vi "Custom - TDD Input Read.vi"(5 "Trigger Offset (dBm)":dbl, 6 "Path Loss (dBm)":dbl, 7 "Sample Count":dbl=16.0, 8 "error in (no error)":errorcluster, 9 "Expected Level (dBm)":dbl, 10 "Center Frequency (MHz)":dbl, 11 "Address":string) -> (0 "error out":errorcluster, 3 "Power":dbl)   [LabVIEW 2025, in "Interface Functions.lvlib"]
uses:
  Interface Functions.lvlib
  <instrlib>/Agilent U2000 Series/Agilent U2000 Series.lvlib
panel:
  out "Commands":string[](array[string])
  # "TDD Input Read"
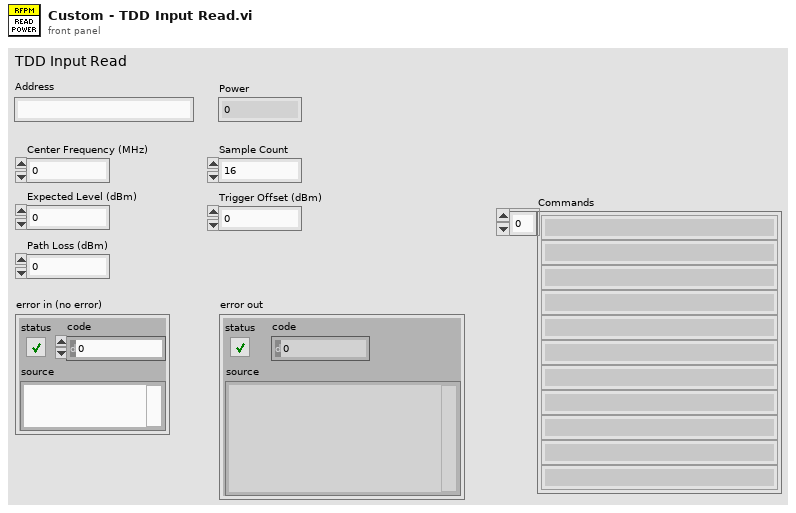
[diagram p1: front panel]
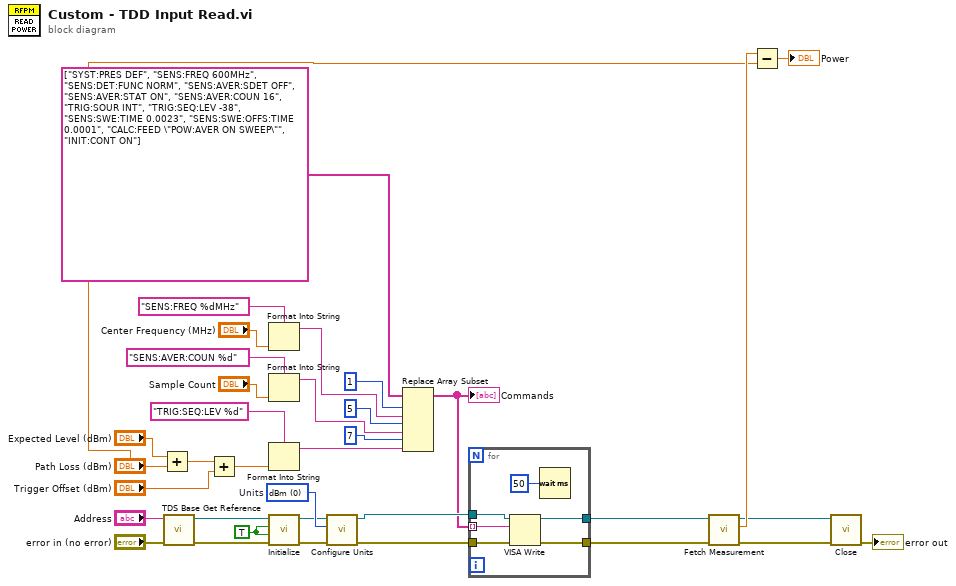
[diagram p0: block diagram]
diagram:
  w26 = u16 0 items=["dBm", "W"]  # Units
  w28 = TRUE ("ID Query (True)")
  n1 = Add(x="Expected Level (dBm)", y="Path Loss (dBm)") -> (x+y=w21:dbl)
  n2 = call "TDS Base Get Reference.vi"("error in (no error)"="error in (no error)", "Address"="Address") -> ("error out"=w31:errorcluster, "Reference"=w29:refnum<visa-resource-name>)  [unwired: 8 in]
  n3 = Add(x=w21, y="Trigger Offset (dBm)") -> (x+y=w8:dbl)
  n4 = Format Into String(format string="SENS:FREQ %dMHz", "Center Frequency (MHz)") -> (resulting string=w13:string)  [unwired: 2 in, 1 out]
  n5 = Format Into String(format string="SENS:AVER:COUN %d", "Sample Count") -> (resulting string=w3:string)  [unwired: 2 in, 1 out]
  n6 = Format Into String(format string="TRIG:SEQ:LEV %d", w8) -> (resulting string=w18:string)  [unwired: 2 in, 1 out]
  n7 = call <instrlib>:"Initialize.vi"("error in (no error)"=w31, "Reset (True)"=w28, "ID Query (True)"=w28, "VISA resource name"=w29) -> ("error out"=w27:errorcluster, "VISA resource name out"=w25:refnum<visa-resource-name>)  [unwired: 6 in]
  n8 = call <instrlib>:"Configure Units.vi"("error in (no error)"=w27, "Units (0: dBm)"=w26, "VISA resource name"=w25) -> ("error out"=w24:errorcluster, "VISA resource name out"=w23:refnum<visa-resource-name>)  [unwired: 1 in, 6 out]
  n9 = Replace Array Subset(array=string[] ["SYST:PRES DEF", "SENS:FREQ 600MHz", "SENS:DET:FUNC NORM", "SENS:AVER:SDET OFF", "SENS:AVER:STAT ON", "SENS:AVER:COUN 16", "TRIG:SOUR INT", "TRIG:SEQ:LEV -38", "SENS:SWE:TIME 0.0023", "SENS:SWE:OFFS:TIME 0.0001", "CALC:FEED \"POW:AVER ON SWEEP\"", "INIT:CONT ON"], new element #1=w13, index #1=1 ("index"), new element #2=w3, index #2=5 ("index"), new element #3=w18, index #3=7 ("index")) -> (w15:string[])
  "Commands" <- w15
  n10 = for {
    tunnel: w15 -> [w41] mode=indexing
    tunnel: [w40] -> w1
    tunnel: [w39] -> w12
    tunnel: w24 -> [w38]
    tunnel: w23 -> [w37]
    n11 = VISA Write(VISA resource name=w37, write buffer=w41, error in (no error)=w38) -> (VISA resource name out=w39:refnum<visa-resource-name>, error out=w40:errorcluster)  [unwired: 1 out]
    n12 = Wait (ms)(milliseconds to wait=u32 50) -> ()  [unwired: 1 out]
  }
  n13 = call <instrlib>:"Fetch Measurement.vi"("error in (no error)"=w1, "VISA resource name"=w12) -> ("error out"=w9:errorcluster, "Measurement"=w11:dbl, "VISA resource name out"=w10:refnum<visa-resource-name>)  [unwired: 7 in]
  n14 = Subtract(x=w11, y="Path Loss (dBm)") -> (x-y=→"Power":dbl)
  n15 = call <instrlib>:"Close.vi"("error in (no error)"=w9, "VISA resource name"=w10) -> ("error out"=→"error out":errorcluster)  [unwired: 9 in]
